vi "list files in llb libraries.vi"() -> (2 "theirs":path[](array[path]), 3 "ours":path[](array[path]))   [LabVIEW 2022 SP3]
uses:
  e91404ee-d232-40cd-87dc-178cddebe457.vi
  4aea7558-7df1-4bfb-b071-3a866cecdf24.vi
  cebfc4fd-2cb4-4afe-a046-bfea519b4f3a.vi
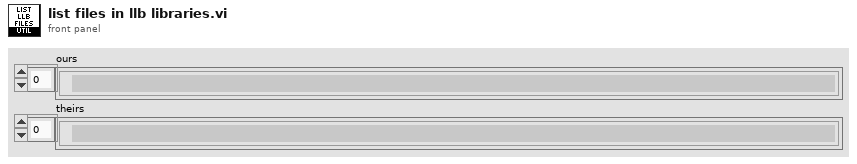
[diagram p1: front panel]
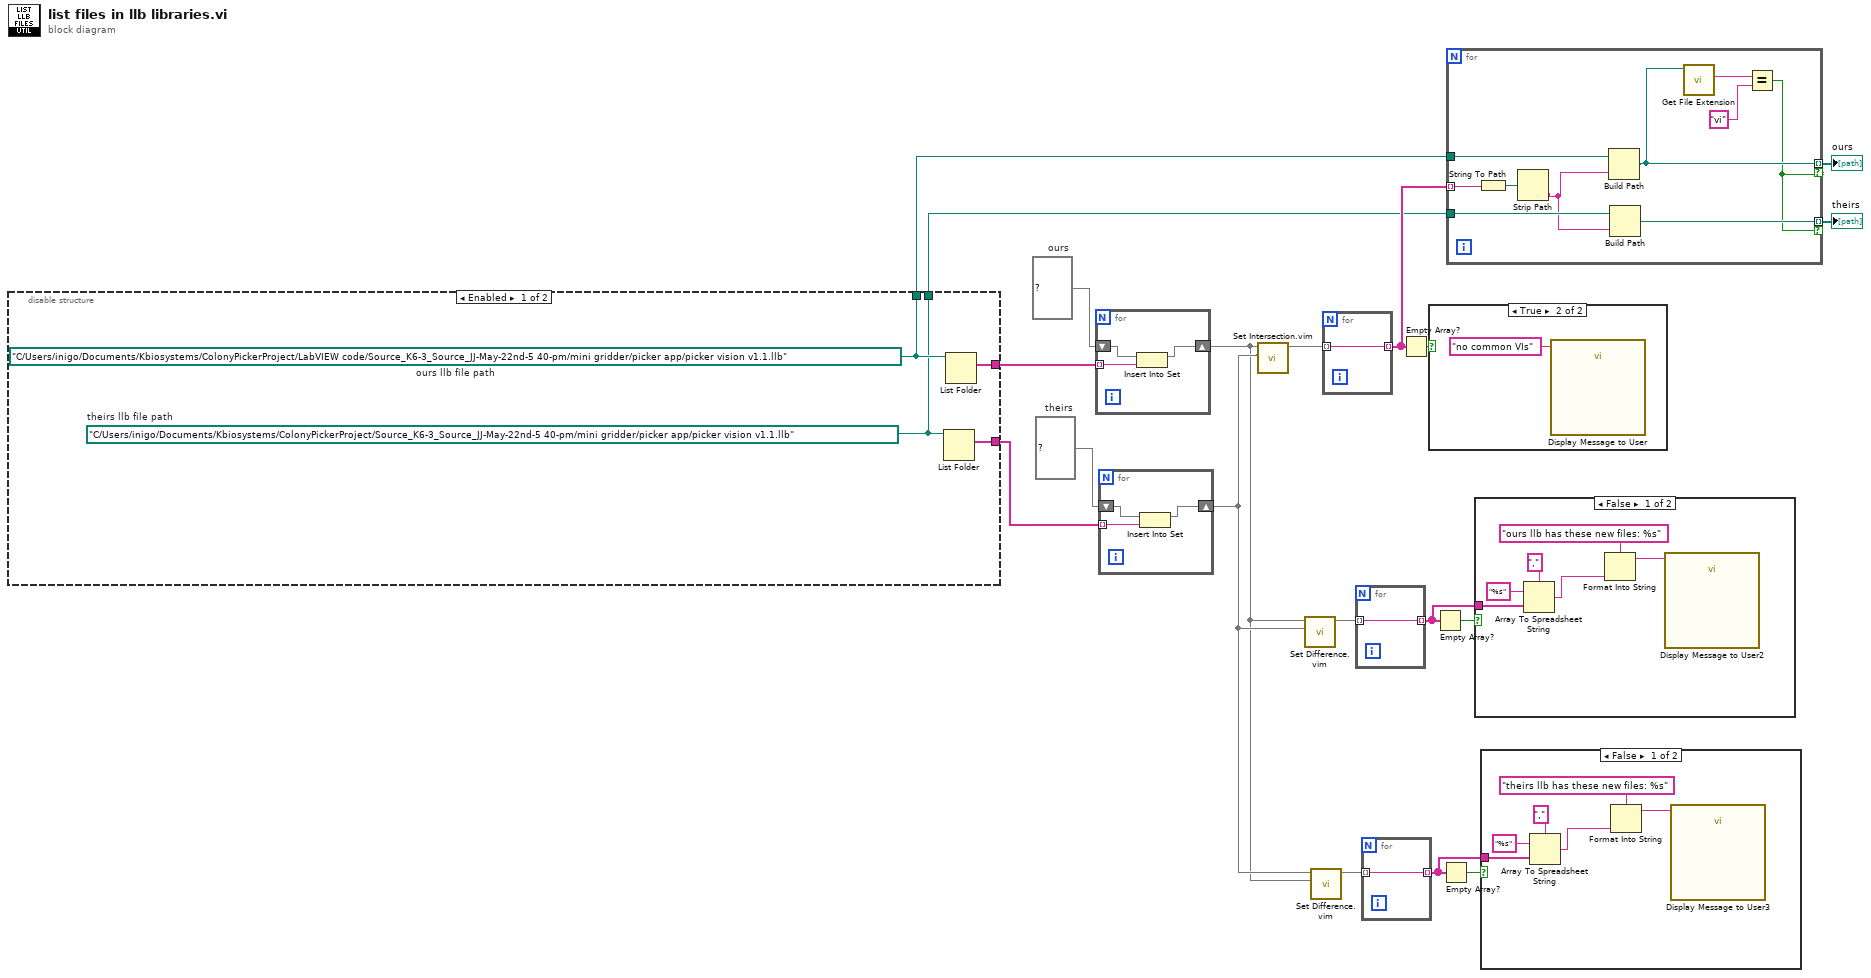
[diagram p0: block diagram]
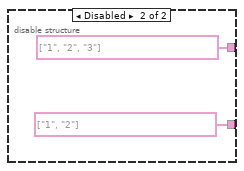
[diagram p2: hidden frame]
diagram:
  w17 = set{string} {}  # theirs
  w18 = set{string} {}  # ours
  n1 = disable-structure shown="Enabled" {
    disable-tunnel: [w23 string[] ["1", "2", "3"] ("filenames")] -> w19
    disable-tunnel: [w22 string[] ["1", "2"] ("filenames")] -> w16
    disable-tunnel: [w21 _] -> w4
    disable-tunnel: [w20 _] -> w3
    frame Enabled {
      w20 = path "C:/Users/inigo/Documents/Kbiosystems/ColonyPickerProject/Source_K6-3_Source_JJ-May-22nd-5 40-pm/mini gridder/picker app/picker vision v1.1.llb"  # theirs llb file path
      w21 = path "C:/Users/inigo/Documents/Kbiosystems/ColonyPickerProject/LabVIEW code/Source_K6-3_Source_JJ-May-22nd-5 40-pm/mini gridder/picker app/picker vision v1.1.llb"  # ours llb file path
      n2 = List Folder(path=w20) -> (filenames=w22:string[])  [unwired: 3 in, 3 out]
      n3 = List Folder(path=w21) -> (filenames=w23:string[])  [unwired: 3 in, 3 out]
    }
    frame Disabled {
    }
  }
  n4 = for {
    tunnel: w19 -> [w28] mode=indexing
    shift-right: [w26] -> w6
    shift-left: w18 -> [w27]
    n5 = Insert Into Set(10:w28, 11:w27) -> (3:w26:set{string})  [unwired: 1 out]
  }
  n6 = for {
    tunnel: w16 -> [w31] mode=indexing
    shift-right: [w29] -> w7
    shift-left: w17 -> [w30]
    n7 = Insert Into Set(10:w31, 11:w30) -> (3:w29:set{string})  [unwired: 1 out]
  }
  n8 = call "Set Intersection.vim"("set 2"=w7, "set 1"=w6) -> ("intersection"=w15:set{string})  [unwired: 9 in]
  n9 = call "Set Difference.vim"("set 2"=w7, "set 1"=w6) -> ("difference"=w13:set{string})  [unwired: 9 in]
  n10 = call "Set Difference.vim"("set 2"=w6, "set 1"=w7) -> ("difference"=w8:set{string})  [unwired: 9 in]
  n11 = for {
    tunnel: [w32] -> w5 mode=indexing
    tunnel: w15 -> [w32] mode=indexing
  }
  n12 = for {
    tunnel: [w33] -> w11 mode=indexing
    tunnel: w13 -> [w33] mode=indexing
  }
  n13 = for {
    tunnel: [w34] -> w10 mode=indexing
    tunnel: w8 -> [w34] mode=indexing
  }
  n14 = Empty Array?(array=w5) -> (empty?=w14:bool)
  n15 = case shown="True" w14 {
    frame False {
    }
    frame True {
      n16 = call "Display Message to User"("Message"="no common VIs") -> ()  [unwired: 9 in, 2 out]
    }
  }
  n17 = Empty Array?(array=w11) -> (empty?=w12:bool)
  n18 = Empty Array?(array=w10) -> (empty?=w9:bool)
  n19 = for {
    tunnel: w5 -> [w45] mode=indexing
    tunnel: w4 -> [w43]
    tunnel: w3 -> [w42]
    tunnel: [w38] -> w2 mode=indexing if=w36
    tunnel: [w37] -> w1 mode=indexing if=w36
    n20 = String To Path(string=w45) -> (path=w44:path)
    n21 = Strip Path(path=w44) -> (name=w41:string)  [unwired: 1 out]
    n22 = Build Path(base path=w43, name or relative path=w41) -> (appended path=w38:path)
    n23 = Build Path(base path=w42, name or relative path=w41) -> (appended path=w37:path)
    n24 = call <vilib>:"Get File Extension.vi"("file"=w38) -> ("lowercase file extension"=w40:string)  [unwired: 6 in, 4 out]
    n25 = Equal?(x=w40, y="vi") -> (x = y?=w36:bool)
  }
  "ours" <- w2
  "theirs" <- w1
  n26 = case shown="False" w12 {
    tunnel: w11 -> [w50 _]
    frame False {
      n27 = Array To Spreadsheet String(delimiter (Tab)=",", array=w50, 3:"%s") -> (spreadsheet string=w47:string)
      n28 = Format Into String(format string="ours llb has these new files: %s", w47) -> (resulting string=w46:string)  [unwired: 2 in, 1 out]
      n29 = call "Display Message to User2"("Message"=w46) -> ()  [unwired: 9 in, 2 out]
    }
    frame True {
    }
  }
  n30 = case shown="False" w9 {
    tunnel: w10 -> [w56 _]
    frame False {
      n31 = Array To Spreadsheet String(delimiter (Tab)=",", array=w56, 3:"%s") -> (spreadsheet string=w53:string)
      n32 = Format Into String(format string="theirs llb has these new files: %s", w53) -> (resulting string=w52:string)  [unwired: 2 in, 1 out]
      n33 = call "Display Message to User3"("Message"=w52) -> ()  [unwired: 9 in, 2 out]
    }
    frame True {
    }
  }
